vi "AddDefaultConfigurationFile.vi"(8 "error in (no error)":errorcluster, 11 "VeriStandTestCase in":refnum<class "VeriStandTestCase.lvclass">) -> (0 "error out":errorcluster, 3 "VeriStandTestCase out":refnum<class "VeriStandTestCase.lvclass">)   [LabVIEW 2027, in "VeriStandTestCase.lvclass"]
uses:
  VeriStandTestCase.lvclass
  VeriStandTestCase.lvclass/VeriStandTestCase.ctl
  <userlib>/_OpenG.lib/file/file.llb/File Exists - Scalar__ogtk.vi
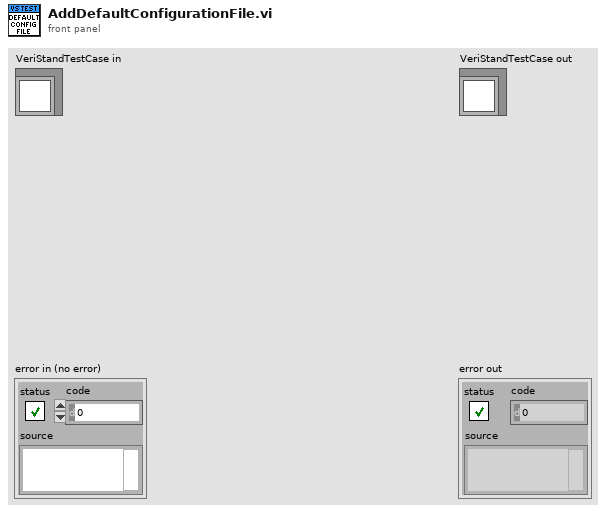
[diagram p1: front panel]
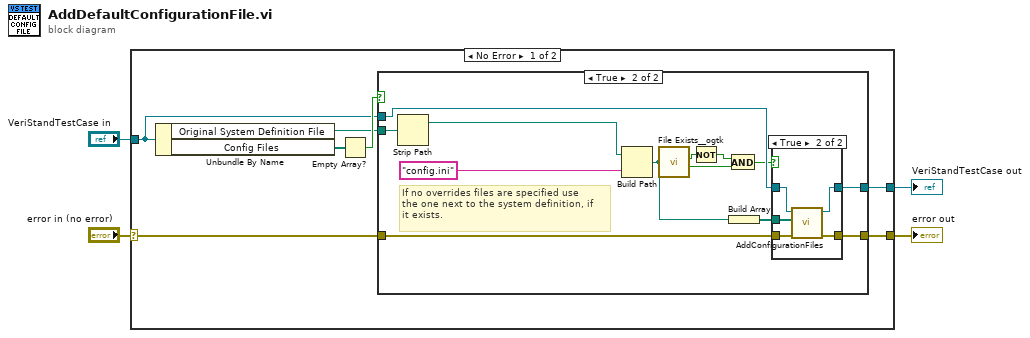
[diagram p0: block diagram]
diagram:
  n1 = case shown="No Error" "error in (no error)" {
    selector: "error in (no error)" -> [w7 w35]
    tunnel: [w6 w35] -> w3
    tunnel: [w8 w34] -> w1
    tunnel: "VeriStandTestCase in" -> [w9 w34]
    frame No Error {
      n2 = Unbundle By Name(w9) -> ("Original System Definition File"=w5:path, "Config Files"=w11:path[])
      n3 = Empty Array?(array=w11) -> (empty?=w10:bool)
      n4 = case shown="True" w10 {
        tunnel: w5 -> [_ w20]
        tunnel: w9 -> [w13 w19]
        tunnel: [w13 w16] -> w8
        tunnel: w7 -> [w12 w15]
        tunnel: [w12 w14] -> w6
        frame False {
        }
        frame True {
          # "If no overrides files are specified use\nthe one next to the system definition, if\nit exists."
          n5 = Strip Path(path=w20) -> (stripped path=w25:path)  [unwired: 1 out]
          n6 = Build Path(base path=w25, name or relative path="config.ini") -> (appended path=w24:path)
          n7 = call-poly <userlib>:"File Exists__ogtk.vi"("file path"=w24) -> ("is directory"=w23:bool, "exists"=w21:bool)  [unwired: 6 in]
          n8 = Not(x=w23) -> (.not. x?=w22:bool)
          n9 = And(x=w22, y=w21) -> (x .and. y?=w18:bool)
          n10 = Build Array(w24) -> (w17:path[])
          n11 = case shown="True" w18 {
            tunnel: w19 -> [w27 w33]
            tunnel: w17 -> [_ w32]
            tunnel: [w27 w31] -> w16
            tunnel: w15 -> [w28 w30]
            tunnel: [w28 w29] -> w14
            frame False {
            }
            frame True {
              n12 = call "AddConfigurationFiles.vi"("error in (no error)"=w30, "configuration files"=w32, "VeriStandTestCase in"=w33) -> ("error out"=w29:errorcluster, "VeriStandTestCase out"=w31:refnum<class "VeriStandTestCase.lvclass">)  [unwired: 7 in]
            }
          }
        }
      }
    }
    frame Error {
    }
  }
  "error out" <- w3
  "VeriStandTestCase out" <- w1
